vi "Write Sender.vi"(10 "Sender":refnum<class "Sender.lvclass">, 11 "Finish Msg in":refnum<class "Finish Msg.lvclass">) -> (3 "Finish Msg out":refnum<class "Finish Msg.lvclass">)   [LabVIEW 2025, in "jettl.lvlib" / "Finish Msg.lvlib" / "Finish Msg.lvclass"]
uses:
  Finish Msg.lvclass
  Finish Msg.lvclass/Finish Msg.ctl
  Sender/Sender/Sender.lvclass
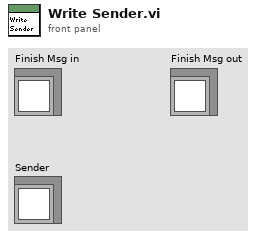
[diagram p1: front panel]
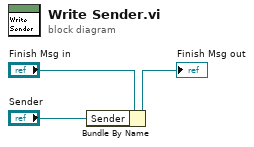
[diagram p0: block diagram]
diagram:
  n1 = Bundle By Name(cluster="Finish Msg in", "Sender"="Sender") -> (→"Finish Msg out":refnum<class "Finish Msg.lvclass">)
